vi "Seq_Start.vi"(8 "error in (no error)":errorcluster, 11 "Qbus in":refnum<class "Qbus.lvclass">) -> (0 "error out":errorcluster)   [LabVIEW 2016, in "SeqProcessor.lvlib"]
uses:
  SeqProcessor.lvlib
  <vilib>/addons/Qbus/Qbus.lvclass
  controls/StepIndex.ctl
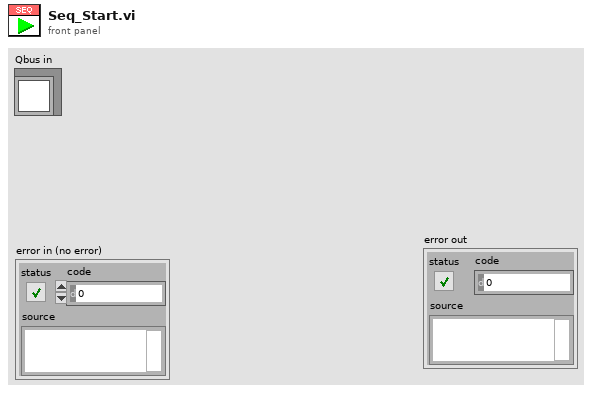
[diagram p1: front panel]
types:
  T1 = typedef "SeqProcessor.lvlib/StepIndex.ctl" = cluster{"Index1":u32, "Index2":u32}
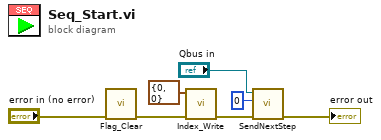
[diagram p0: block diagram]
diagram:
  n1 = call "Flag_Clear.vi"("error in (no error)"="error in (no error)") -> ("error out"=w2:errorcluster)  [unwired: 10 in]
  n2 = call "Index_Write.vi"("error in (no error)"=w2, "Index"=T1 {"Index1"=0, "Index2"=0}) -> ("error out"=w4:errorcluster)  [unwired: 9 in]
  n3 = call "SendNextStep.vi"("error in (no error)"=w4, "StepIndex"=u32 0, "Qbus in"="Qbus in") -> ("error out"=→"error out":errorcluster)  [unwired: 8 in]
